vi "Priority Convert.vi"(10 "Priority":bool) -> (2 "Priority":T1)   [LabVIEW 2025, in "jettl.lvlib" / "Transport.lvlib" / "Event Transport.lvclass"]
uses:
  Transport/Event Transport/Event Transport.lvclass
  Transport/Event Transport/Event Transport.lvclass/Event Transport.ctl
  <vilib>/event_ctls.llb/usereventprio.ctl
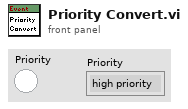
[diagram p1: front panel]
types:
  T1 = typedef "usereventprio.ctl" = enum32{"high priority", "normal priority"}
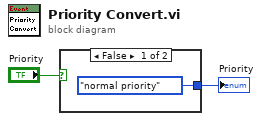
[diagram p0: block diagram]
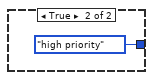
[diagram p2: hidden frame]
diagram:
  n1 = case shown="False" "Priority" {
    tunnel: [usereventprio."normal priority" ("priority (normal)") usereventprio."high priority" ("priority (normal)")] -> w1
    frame False {
    }
    frame True {
    }
  }
  "Priority" <- w1
